vi "write TBM configuration.vi"(8 "error in":errorcluster, 10 "configuration":refnum<class "TBM configuration.lvclass">, 11 "module editor node in":refnum<class "module editor node.lvclass">) -> (0 "error out":errorcluster, 3 "module editor node out":refnum<class "module editor node.lvclass">)   [LabVIEW 2013, in "PL Framework Configuration Tool.lvlib" / "module editor node.lvclass"]
uses:
  module editor node.lvclass
  <vilib>/NI/Tag Bus Module Framework/root configuration/TBM configuration.lvclass
  TBM Configuration Node/TBM Configuration Node.lvclass
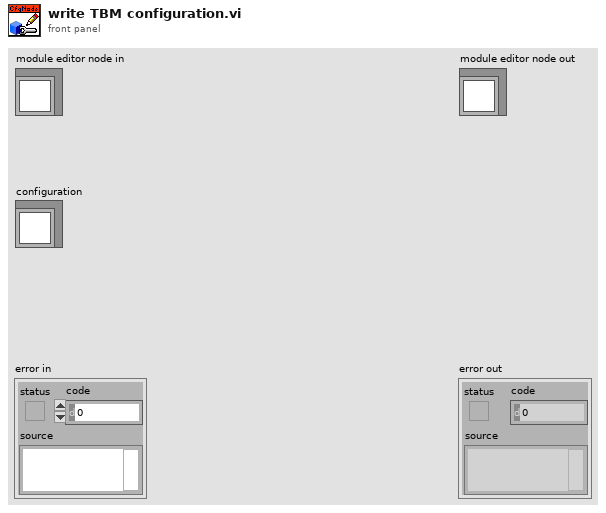
[diagram p1: front panel]
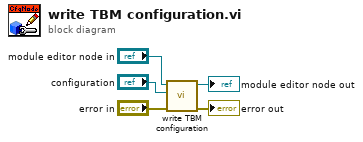
[diagram p0: block diagram]
diagram:
  n1 = call-parent "write TBM configuration.vi"("error in"="error in", "configuration"="configuration", "TBM Configuration Node in"="module editor node in") -> ("error out"=→"error out":errorcluster, "TBM Configuration Node out"=→"module editor node out":refnum<class "module editor node.lvclass">)  [unwired: 7 in]
